vi "Start read modules.vi"(7 "N_moduls":i32, 8 "error in":errorcluster, 10 "Param Referense":T1, 11 "classes":refnum<class "MB_TCP.lvclass">[](array[class])) -> (0 "error out":errorcluster)   [LabVIEW 2019, in "MB_TCP.lvclass"]
uses:
  MB_TCP.lvclass
  ICPCON Param/ICPCON Param.ctl
  ICPCON Param/Eth timeouts.ctl
  MB timeouts.ctl
  NI_modbus_upd/TCP/tcp timeouts.ctl
  MB_TCP.lvclass/MB_TCP.ctl
  NI_modbus_upd/TCP/TCP.lvclass/TCP.ctl
  Execute.vi
  ICPCON Param/ICPCON_Param.lvlib
  NI_modbus_upd/TCP/TCP.lvclass
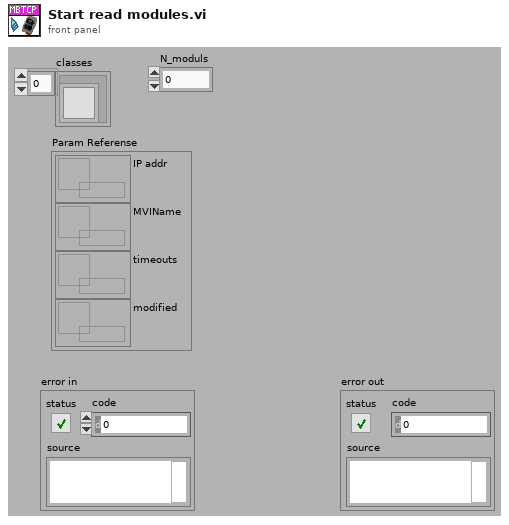
[diagram p1: front panel]
types:
  T1 = typedef "ICPCON_Param.lvlib/ICPCON Param.ctl" = cluster{"IP addr":refnum<data-value>, "MVIName":refnum<data-value>, "timeouts":refnum<data-value>, "modified":refnum<data-value>}
  T2 = typedef "TCP.lvclass/tcp timeouts.ctl" = cluster{"connect timeout":i32, "write timeout":i32, "read timeout":i32}
  T3 = typedef "MB_TCP.lvclass/MB timeouts.ctl" = cluster{"reconn_timeout":i32, "N attempt max":i32, "t_reset_TTL":i32, "period":i32}
  T4 = typedef "ICPCON_Param.lvlib/Eth timeouts.ctl" = cluster{"conn_timeout":i32, "reconn_timeout":i32, "N attempt max":i32, "t_reset_TTL":i32, "write_timeout":i32, "read_timeout":i32, "period":i32}
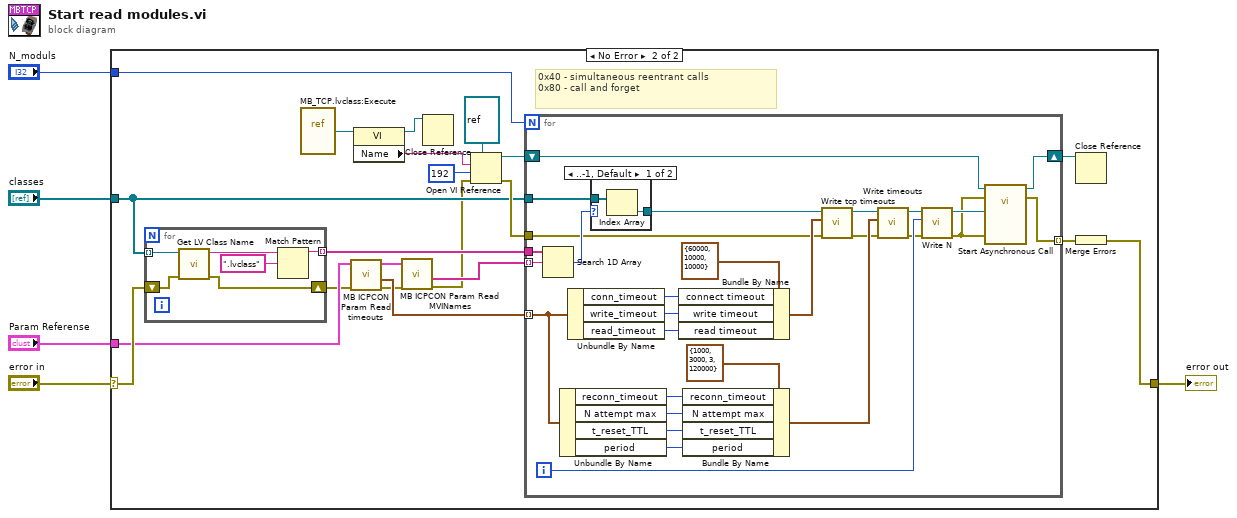
[diagram p0: block diagram]
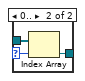
[diagram p3: hidden frame]
diagram:
  n1 = case shown="No Error" "error in" {
    selector: "error in" -> [w6 w13]
    tunnel: "N_moduls" -> [_ w22]
    tunnel: [w6 w26] -> w5
    tunnel: "Param Referense" -> [_ w12]
    tunnel: "classes" -> [_ w14]
    frame Error {
    }
    frame No Error {
      # "0x40 - simultaneous reentrant calls\n0x80 - call and forget"
      n2 = for {
        tunnel: w14 -> [w33] mode=indexing
        tunnel: [w29] -> w15 mode=indexing
        shift-right: [w32] -> w9
        shift-left: w13 -> [w28]
        n3 = call <vilib>:"Get LV Class Name.vi"("error in (no error)"=w28, "object"=w33) -> ("error out"=w32:errorcluster, "class name"=w31:string)  [unwired: 8 in]
        n4 = Match Pattern(string=w31, regular expression=".lvclass") -> (before substring=w29:string)  [unwired: 1 in, 3 out]
      }
      n5 = vi-ref "MB_TCP.lvclass:Execute.vi"() -> (w25:refnum<vi>)
      n6 = call "MB ICPCON Param Read timeouts.vi"("error in (no error)"=w9, "Param Reference in"=w12) -> ("error out"=w10:errorcluster, "timeouts"=w24:T4[], "Param Reference out"=w11:T1)  [unwired: 7 in]
      n7 = property class="VI"(reference=w25) -> (reference out=w21:refnum<vi>, "Name"=w19:string)  [unwired: 1 in, 1 out]
      n8 = call "MB ICPCON Param Read MVINames.vi"("error in (no error)"=w10, "Param Reference in"=w11) -> ("error out"=w8:errorcluster, "MVIName"=w23:string[])  [unwired: 7 in, 1 out]
      n9 = Close Reference(reference=w21) -> ()  [unwired: 1 in, 1 out]
      n10 = Open VI Reference(type specifier VI Refnum (for type only)=refnum<vi> refnum, vi path=w19, options=192, error in (no error)=w8) -> (vi reference=w17:refnum<vi>, error out=w18:errorcluster)  [unwired: 2 in]
      n11 = for {
        N: w22 -> [_]
        tunnel: [w61] -> w27 mode=indexing
        tunnel: w24 -> [w40] mode=indexing
        tunnel: w23 -> [w50] mode=indexing
        tunnel: w14 -> [w60]
        tunnel: w15 -> [w59]
        tunnel: w18 -> [w35]
        shift-right: [w48] -> w7
        shift-left: w17 -> [w49]
        i -> [w51]
        n12 = Search 1D Array(1D array=w59, element=w50) -> (index of element=w58:i32)  [unwired: 1 in]
        n13 = Unbundle By Name(w40) -> ("reconn_timeout"=w56:i32, "N attempt max"=w55:i32, "t_reset_TTL"=w54:i32, "period"=w53:i32)
        n14 = Unbundle By Name(w40) -> ("conn_timeout"=w43:i32, "write_timeout"=w42:i32, "read_timeout"=w41:i32)
        n15 = case shown="..-1, Default" w58 {
          selector: w58 -> [_ w64]
          tunnel: w60 -> [w63 w66]
          tunnel: [w62 w65] -> w34
          frame ..-1, Default {
            n16 = Index Array(array=w63) -> (element=w62:refnum<class "MB_TCP.lvclass">)  [unwired: 1 in]
          }
          frame 0.. {
            n17 = Index Array(array=w66, index=w64) -> (element=w65:refnum<class "MB_TCP.lvclass">)
          }
        }
        n18 = Bundle By Name(cluster=T2 {"connect timeout"=60000, "write timeout"=10000, "read timeout"=10000} ("tcp timeouts"), "connect timeout"=w43, "write timeout"=w42, "read timeout"=w41) -> (w39:T2)
        n19 = Bundle By Name(cluster=T3 {"reconn_timeout"=1000, "N attempt max"=3000, "t_reset_TTL"=3, "period"=120000} ("timeouts"), "reconn_timeout"=w56, "N attempt max"=w55, "t_reset_TTL"=w54, "period"=w53) -> (w52:T3)
        n20 = call "Write tcp timeouts.vi"("error in (no error)"=w35, "tcp timeouts"=w39, "MB_TCP in"=w34) -> ("error out"=w37:errorcluster, "MB_TCP out"=w38:refnum<class "MB_TCP.lvclass">)  [unwired: 7 in]
        n21 = call "Write timeouts.vi"("error in (no error)"=w37, "MB timeouts"=w52, "MB_TCP in"=w38) -> ("error out"=w46:errorcluster, "MB_TCP out"=w45:refnum<class "MB_TCP.lvclass">)  [unwired: 7 in]
        n22 = call "Write N.vi"("error in (no error)"=w46, "N"=w51, "MB_TCP in"=w45) -> ("error out"=w36:errorcluster, "MB_TCP out"=w47:refnum<class "MB_TCP.lvclass">)  [unwired: 7 in]
        n23 = call-by-ref "Start Asynchronous Call"(reference=w49, error in=w36, 8:"error in (no error)"=w36, "MB_TCP in"=w47) -> (reference out=w48:refnum<vi>, error out=w61:errorcluster)  [unwired: 7 in, 3 out]
      }
      n24 = Close Reference(reference=w7) -> ()  [unwired: 1 in, 1 out]
      n25 = Merge Errors(w27) -> (w26:errorcluster)
    }
  }
  "error out" <- w5
